vi "2810A Initial Connect Multiple.vi"(8 "error in (no error)":errorcluster, 10 "JSONCluster":T1, 11 "IVI Refnum in":refnum<k15>) -> (0 "error out":errorcluster, 2 "Scan List Channels":string[](array[string]), 3 "IVI Refnum out":refnum<k15>)   [LabVIEW 2019, in "SupportVIs.lvlib"]
uses:
  SupportVIs.lvlib
  JSONCluster.ctl
  <instrlib>/niSwitch/niSwitch.llb/niSwitch Connect Channels (Multiple).vi
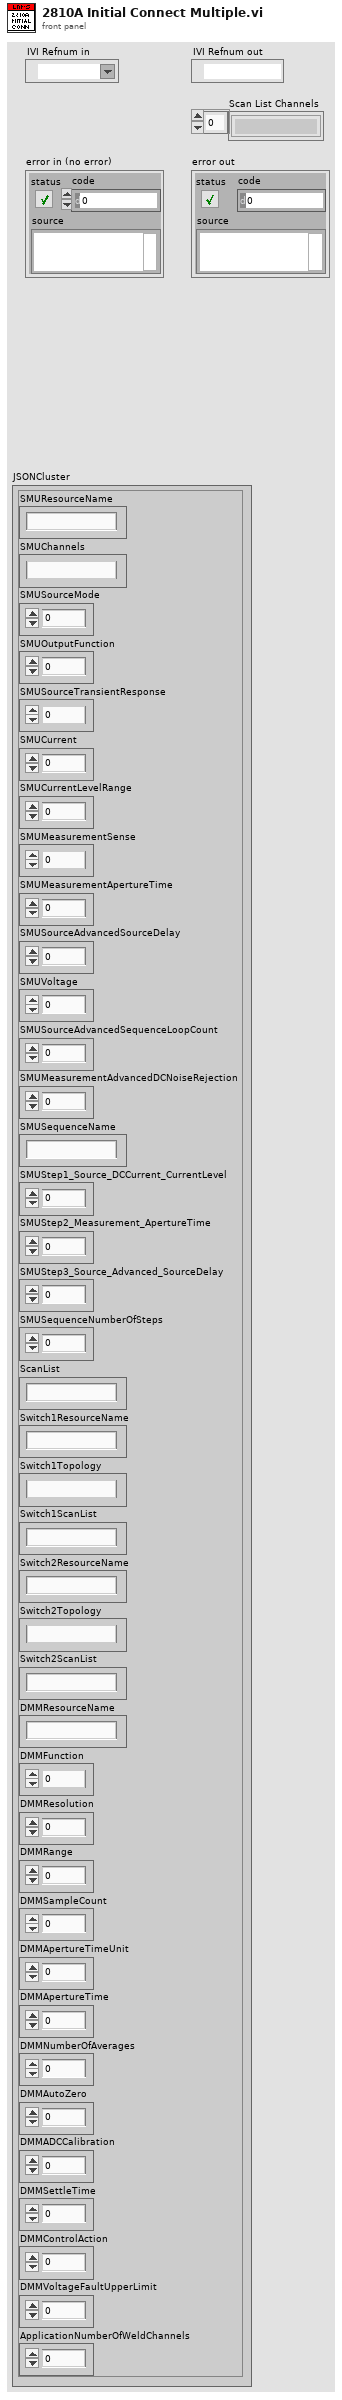
[diagram p1: front panel]
types:
  T1 = typedef "JSONCluster.ctl" = cluster{"SMUResourceName":string, "SMUChannels":string, "SMUSourceMode":i32, "SMUOutputFunction":i32, "SMUSourceTransientResponse":i32, "SMUCurrent":dbl, "SMUCurrentLevelRange":dbl, "SMUMeasurementSense":i32, "SMUMeasurementApertureTime":dbl, "SMUSourceAdvancedSourceDelay":dbl, "SMUVoltage":dbl, "SMUSourceAdvancedSequenceLoopCount":i32, "SMUMeasurementAdvancedDCNoiseRejection":i32, "SMUSequenceName":string, "SMUStep1_Source_DCCurrent_CurrentLevel":i32, "SMUStep2_Measurement_ApertureTime":i32, "SMUStep3_Source_Advanced_SourceDelay":i32, "SMUSequenceNumberOfSteps":i32, "ScanList":string, "Switch1ResourceName":string, "Switch1Topology":string, "Switch1ScanList":string, "Switch2ResourceName":string, "Switch2Topology":string, "Switch2ScanList":string, "DMMResourceName":string, "DMMFunction":i32, "DMMResolution":dbl, "DMMRange":dbl, "DMMSampleCount":i32, "DMMApertureTimeUnit":i32, "DMMApertureTime":dbl, "DMMNumberOfAverages":i32, "DMMAutoZero":i32, "DMMADCCalibration":i32, "DMMSettleTime":dbl, "DMMControlAction":i32, "DMMVoltageFaultUpperLimit":dbl, "ApplicationNumberOfWeldChannels":i32}
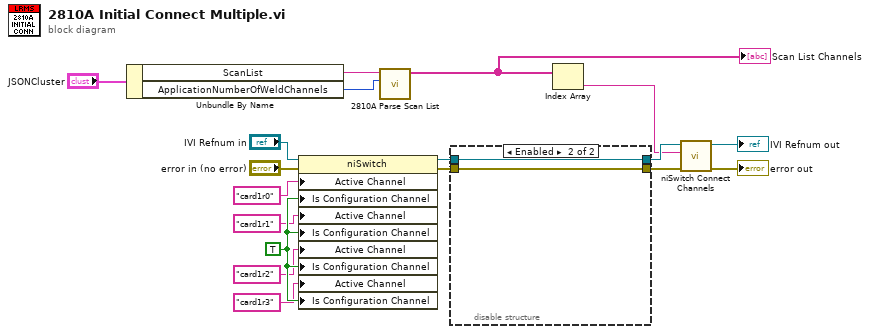
[diagram p0: block diagram]
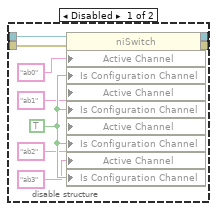
[diagram p2: hidden frame]
diagram:
  w12 = TRUE ("Channel Configuration:Is Source Channel")
  n1 = Unbundle By Name("JSONCluster") -> ("ScanList"=w3:string, "ApplicationNumberOfWeldChannels"=w1:i32)
  n2 = property class="niSwitch"(reference="IVI Refnum in", error in="error in (no error)", "Active Channel"="card1r0", "Is Configuration Channel"=w12, "Active Channel"="card1r1", "Is Configuration Channel"=w12, "Active Channel"="card1r2", "Is Configuration Channel"=w12, "Active Channel"="card1r3", "Is Configuration Channel"=w12) -> (reference out=w15:refnum<k15>, error out=w16:errorcluster)
  n3 = call "2810A Parse Scan List.vi"("ApplicationNumberOfWeldChannels"=w1, "Matrix Input String"=w3) -> ("Channel Array"=w2:string[])  [unwired: 9 in]
  "Scan List Channels" <- w2
  n4 = disable-structure shown="Enabled" {
    disable-tunnel: [w22 w28] -> w18
    disable-tunnel: [w21 w29] -> w17
    disable-tunnel: w16 -> [w20 w28]
    disable-tunnel: w15 -> [w19 w29]
    frame Disabled {
      w27 = TRUE ("Channel Configuration:Analog Bus Sharing Enable")
      n5 = property class="niSwitch"(reference=w19, error in=w20, "Active Channel"="ab0", "Is Configuration Channel"=w27, "Active Channel"="ab1", "Is Configuration Channel"=w27, "Active Channel"="ab2", "Is Configuration Channel"=w27, "Active Channel"="ab3", "Is Configuration Channel"=w27) -> (reference out=w21:refnum<k15>, error out=w22:errorcluster)
    }
    frame Enabled {
    }
  }
  n6 = Index Array(array=w2) -> (element=w5:string)  [unwired: 1 in]
  n7 = call-poly <instrlib>:"niSwitch Connect Channels.vi"("error in (no error)"=w18, "connection list"=w5, "instrument handle"=w17) -> ("error out"=→"error out":errorcluster, "instrument handle out"=→"IVI Refnum out":refnum<k15>)  [unwired: 7 in]
